vi "Split_Data_Test.vi"() -> ()   [LabVIEW 2023]
uses:
  <vilib>/Analysis/2dsp.llb/1D Cross Correlation (DBL).vi
  <vilib>/measure/NI_MABase.lvlib
  <vilib>/Analysis/NI_AALPro.lvlib
panel:
  out "Split_Queue4":string
  out "Split_Queue4_Result":string[](array[string])
  out "Split_Queue3_Result":string[](array[string])
  out "Split_Queue2_Result":string[](array[string])
  out "Split_Queue3":string
  out "Split_Queue2":string
  out "연결된 문자열 5":string
  out "연결된 문자열 4":string
  out "연결된 문자열 3":string
  out "연결된 문자열 2":string
  out "웨이브폼 그래프":waveform(dbl)(graph)
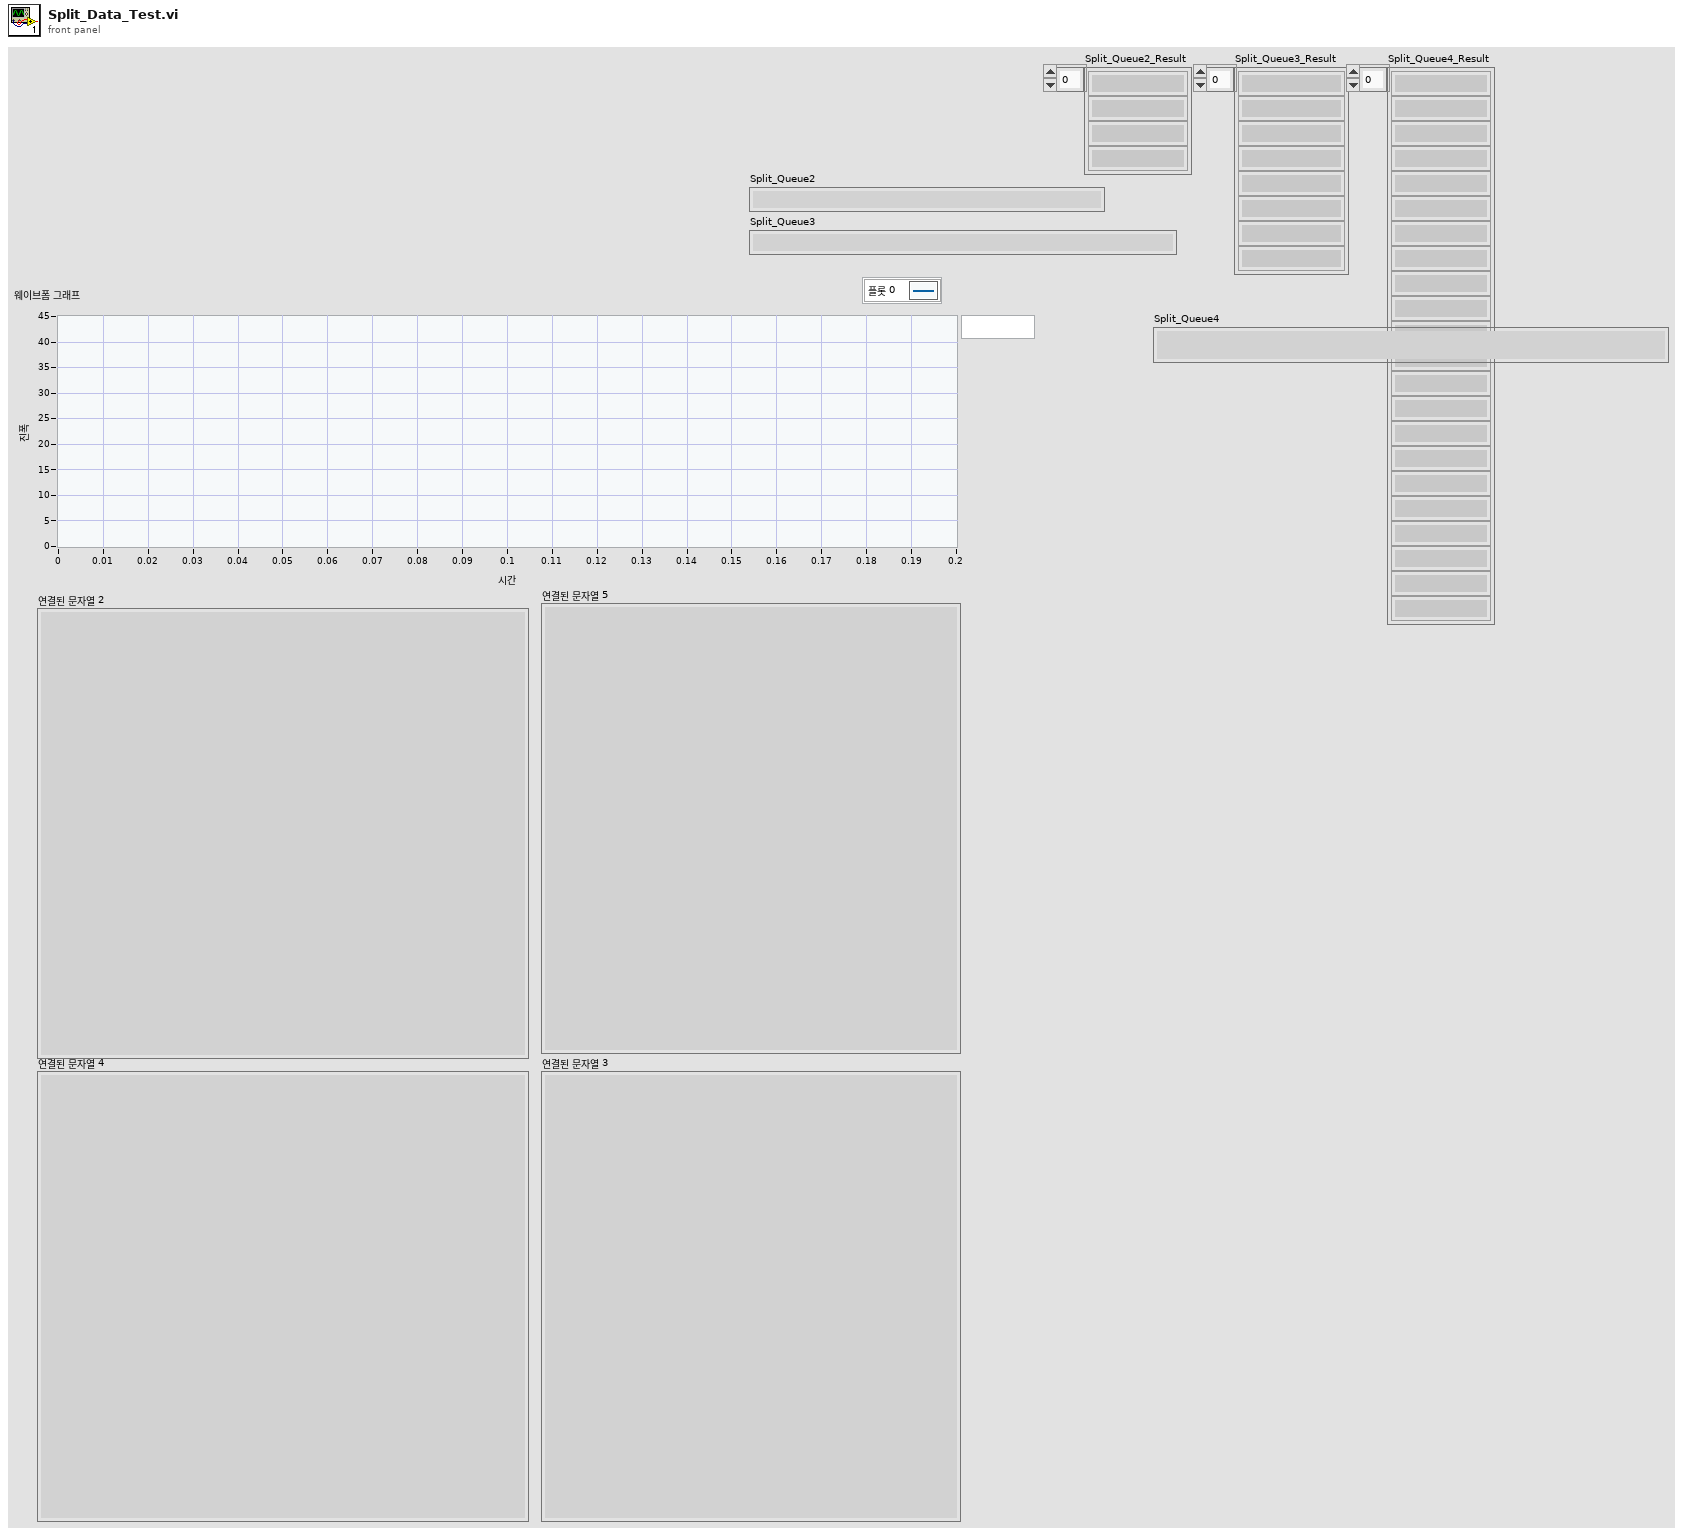
[diagram p1: front panel]
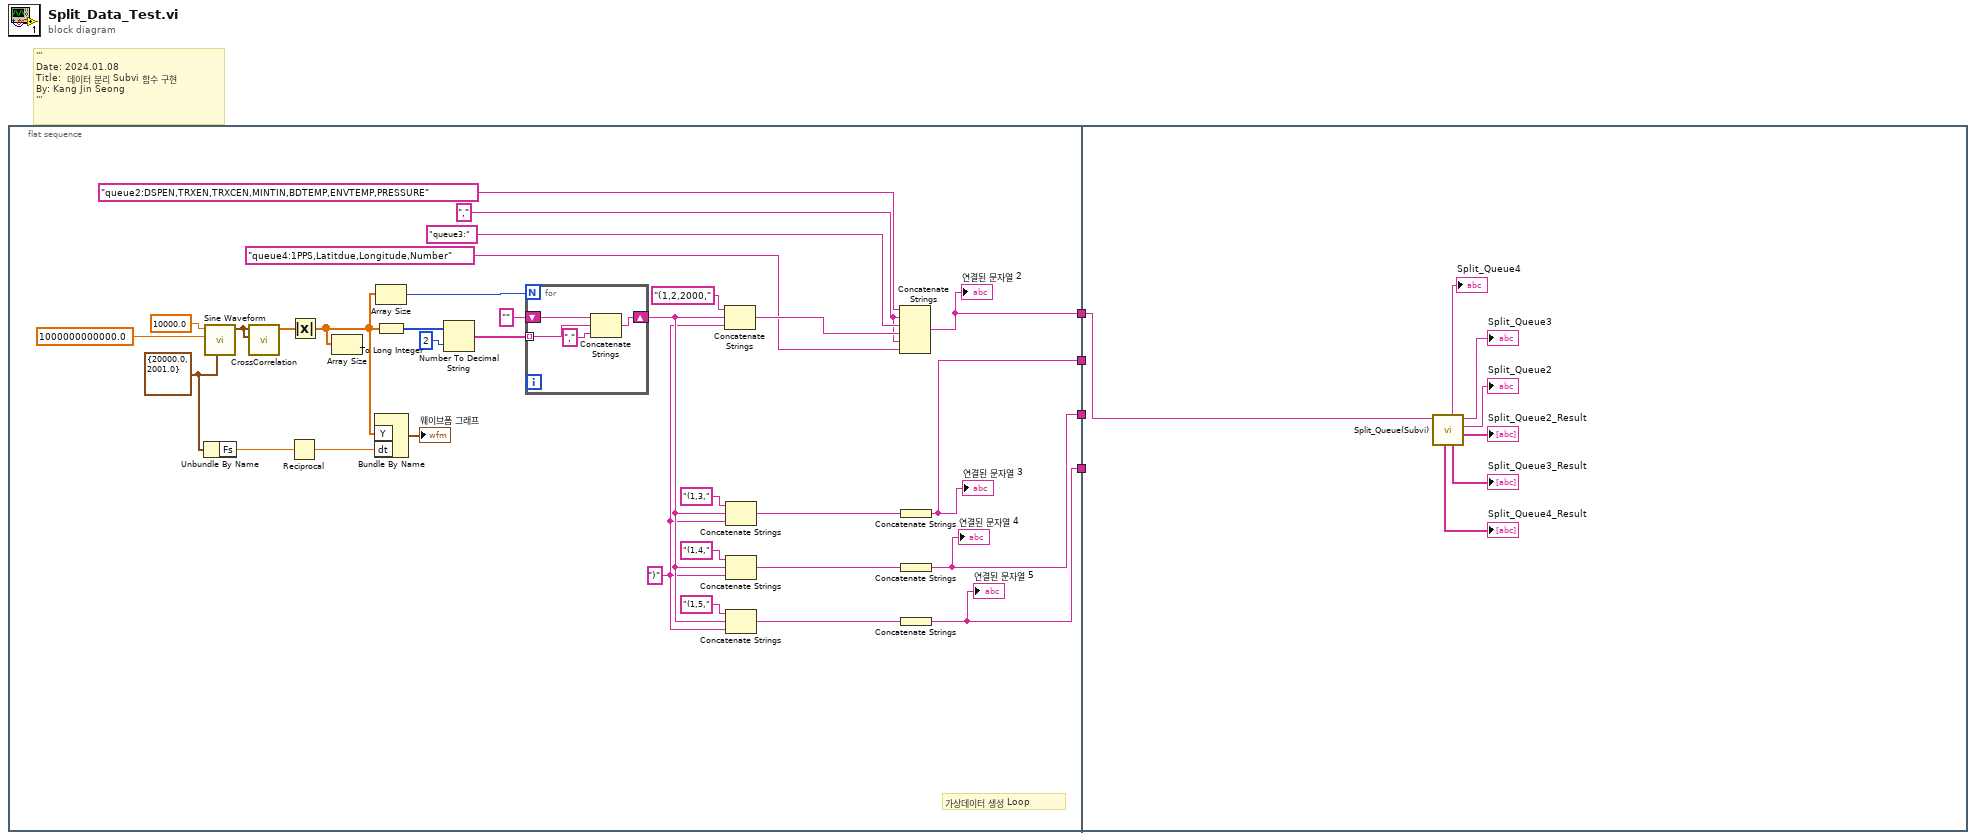
[diagram p0: block diagram]
diagram:
  # "'''\nDate: 2024.01.08\nTitle:  데이터 분리 Subvi 함수 구현\nBy: Kang Jin Seong\n'''"
  n1 = flat-sequence {
    tunnel: [w13] -> w4
    tunnel: [w12] -> w3
    tunnel: [w11] -> w2
    tunnel: [w10] -> w1
    tunnel: w4 -> [w42]
    tunnel: w3 -> [_]
    tunnel: w2 -> [_]
    tunnel: w1 -> [_]
    frame #0 {
      w6 = ","
      w17 = ")"
      w34 = cluster{"Fs":dbl, "#s":dbl} {"Fs"=20000.0, "#s"=2001.0} ("sampling info")
      # "가상데이터 생성 Loop"
      n2 = Unbundle By Name(w34) -> ("Fs"=w33:dbl)
      n3 = call <vilib>:"Sine Waveform.vi"("sampling info"=w34, "amplitude"=1000000000000.0, "frequency"=10000.0) -> ("signal out"=w35:waveform(dbl))  [unwired: 7 in, 1 out]
      n4 = call-poly <vilib>:"CrossCorrelation.vi"("Y"=w35, "X"=w35) -> ("Rxy"=w30:dbl[])  [unwired: 8 in, 1 out]
      n5 = Reciprocal(x=w33) -> (1/x=w32:dbl)
      n6 = Absolute Value(x=w30) -> (abs(x)=w26:dbl[])
      n7 = Array Size(array=w26) -> ()  [unwired: 1 out]
      n8 = Bundle By Name("Y"=w26, "dt"=w32) -> (→"웨이브폼 그래프":waveform(dbl))  [unwired: 1 in]
      n9 = Array Size(array=w26) -> (size(s)=w28:i32)
      n10 = To Long Integer(number=w26) -> (32bit integer=w25:i32[])
      n11 = Number To Decimal String(number=w25, width (-)=i16 2 ("폭(-)")) -> (decimal integer string=w23:string[])
      n12 = for {
        N: w28 -> [_]
        shift-right: [w39] -> w18
        shift-left: "" -> [w40]
        tunnel: w23 -> [w38] mode=indexing
        n13 = Concatenate Strings(w40, w38, ",") -> (w39:string)
      }
      n14 = Concatenate Strings("(1,2,2000,", w18, w17) -> (w7:string)
      n15 = Concatenate Strings("(1,3,", w18, w17) -> (w16:string)
      n16 = Concatenate Strings("(1,4,", w18, w17) -> (w15:string)
      n17 = Concatenate Strings("(1,5,", w18, w17) -> (w14:string)
      n18 = Concatenate Strings("queue2:DSPEN,TRXEN,TRXCEN,MINTIN,BDTEMP,ENVTEMP,PRESSURE", w6, "queue3:", w7, w6, "queue4:1PPS,Latitdue,Longitude,Number") -> (w13:string)
      "연결된 문자열 2" <- w13
      n19 = Concatenate Strings(w16) -> (w12:string)
      "연결된 문자열 3" <- w12
      n20 = Concatenate Strings(w15) -> (w11:string)
      "연결된 문자열 4" <- w11
      n21 = Concatenate Strings(w14) -> (w10:string)
      "연결된 문자열 5" <- w10
    }
    frame #1 {
      n22 = call "Split_Queue(Subvi).vi"("입력 문자열"=w42) -> ("Split_Queue2_Result"=→"Split_Queue2_Result":string[], "Split_Queue2"=→"Split_Queue2":string, "Split_Queue3"=→"Split_Queue3":string, "Split_Queue3_Result"=→"Split_Queue3_Result":string[], "Split_Queue4"=→"Split_Queue4":string, "Split_Queue4_Result"=→"Split_Queue4_Result":string[])  [unwired: 5 in]
    }
  }
